vi "SCCSup Lock VI.vi"(4 "error in (no error)":errorcluster, 7 "reference":refnum<vi>) -> (0 "error out":errorcluster, 3 "reference out":refnum<vi>)   [LabVIEW 2017]
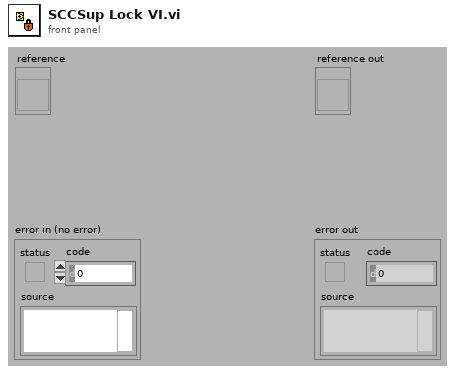
[diagram p1: front panel]
types:
  T1 = enum32{"invalid lock state", "Not Locked", "Locked (No Password)", "Password-protected"}
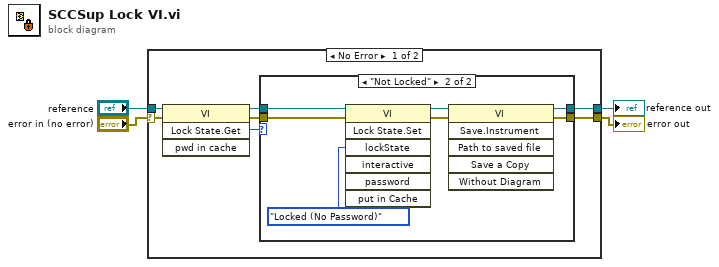
[diagram p0: block diagram]
diagram:
  n1 = case shown="No Error" "error in (no error)" {
    selector: "error in (no error)" -> [w8 w22]
    tunnel: [w6 w22] -> w4
    tunnel: "reference" -> [w7 w21]
    tunnel: [w5 w21] -> w1
    frame No Error {
      n2 = invoke class="VI" method="Lock State.Get"(reference=w7, error in=w8) -> (reference out=w11:refnum<vi>, error out=w10:errorcluster, "Get Lock State"=w9:T1)  [unwired: 2 in, 1 out]
      n3 = case shown="\"Not Locked\"" w9 {
        tunnel: w11 -> [w13 w20]
        tunnel: w10 -> [w12 w19]
        tunnel: [w13 w14] -> w5
        tunnel: [w12 w15] -> w6
        frame Default {
        }
        frame "Not Locked" {
          n4 = invoke class="VI" method="Lock State.Set"(reference=w20, error in=w19, "lockState"=T1."Locked (No Password)") -> (reference out=w17:refnum<vi>, error out=w16:errorcluster)  [unwired: 4 in, 5 out]
          n5 = invoke class="VI" method="Save.Instrument"(reference=w17, error in=w16) -> (reference out=w14:refnum<vi>, error out=w15:errorcluster)  [unwired: 4 in, 4 out]
        }
      }
    }
    frame Error {
    }
  }
  "error out" <- w4
  "reference out" <- w1
